vi "UnexpectedDepsCheck.vi"(6 "GUI Mode? {F)":bool, 8 "error in (no error)":errorcluster, 10 "CheckChangedLibrariesOnly":bool=TRUE, 11 "Workspace Path":path=path "C:/sw-deps-monitor") -> (0 "error out":errorcluster, 2 "Status Indicator":string, 3 "Failures":T1[](array[typedef]))   [LabVIEW 2019, in "DepsWatch.lvlib"]
uses:
  DepsWatch.lvlib
  Typedefs/DepsCheckResult.ctl
  28450a76-a9d3-48c7-9439-369bd691228e.vi
  <vilib>/JDP Science/JSONtext/Variant to JSON Text.vi
  <vilib>/Wiresmith Technology/G CLI/CLI Class/CLI.lvclass
  <vilib>/JDP Science/JSONtext/LVClass Serializer/JSONtext LVClass Serializer.lvclass
  <vilib>/SLL Toolkit/SLL String/SLL String.lvlib
  <vilib>/JDP Science/JSONtext/JSONtext.lvlib
panel:
  in  "Tab Control":enum32{"GUI Mode", "CLI Mode"}(tab)
  out "Args":string[](array[string])=["C:\\sw-deps-monitor", "True"]
  # "When in GUI Mode, the controls will be used, \nIn CLI Mode, the Args will be used"
  # "Workspace Path"
  # "CheckChangedLibrariesOnly? True/False"
  # "Command to run the VI from terminal\ng-cli -v --lv-ver 2023 --arch 32 \"C:\\sw-deps-monitor\\CICD\\AutomatedChecks\\UnexpectedDepsCheck.vi\" -- \"C:\\sw-deps-monitor\" \"False\""
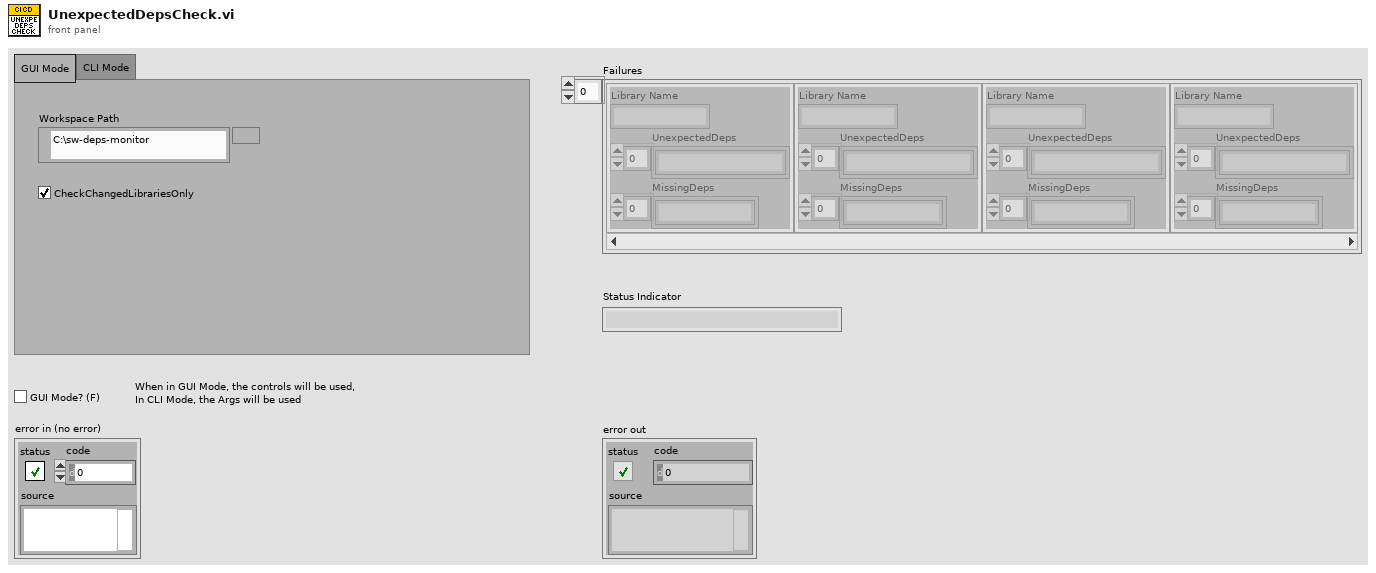
[diagram p1: front panel]
types:
  T1 = typedef "DepsWatch.lvlib/DepsCheckResult.ctl" = cluster{"Library Name":string, "UnexpectedDeps":string[], "MissingDeps":string[]}
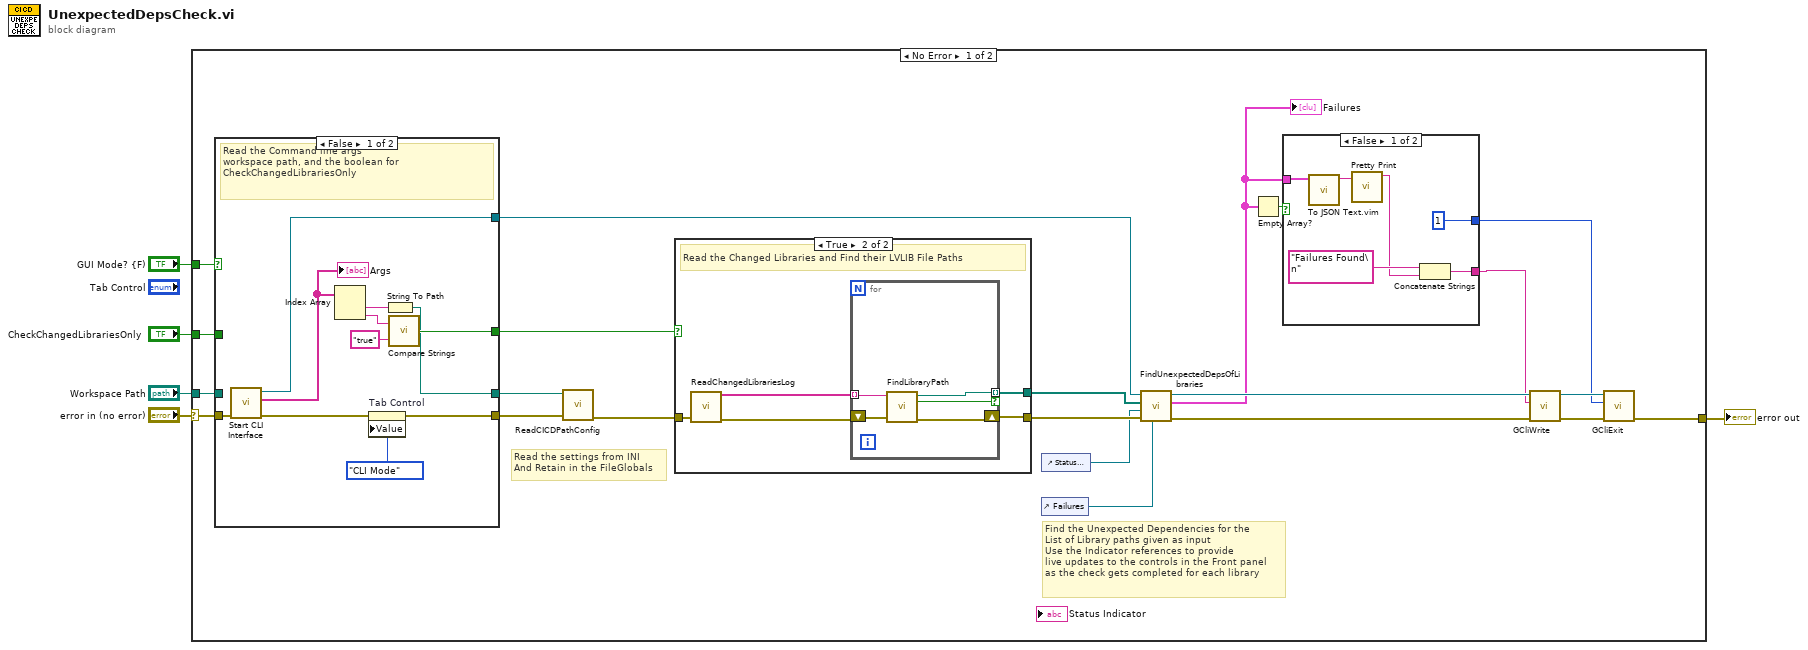
[diagram p0: block diagram]
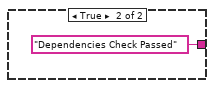
[diagram p2: hidden frame]
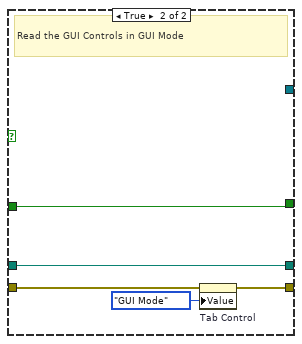
[diagram p3: hidden frame]
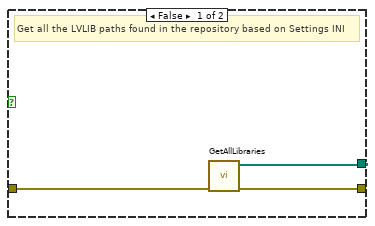
[diagram p4: hidden frame]
diagram:
  n1 = case shown="No Error" "error in (no error)" {
    selector: "error in (no error)" -> [w25 w64]
    tunnel: "GUI Mode? {F)" -> [w26 _]
    tunnel: [w14 w64] -> w3
    tunnel: "CheckChangedLibrariesOnly" -> [w8 _]
    tunnel: "Workspace Path" -> [w7 _]
    frame No Error {
      # "Find the Unexpected Dependencies for the\nList of Library paths given as input\nUse the Indicator references to provide \nlive updates to the controls in the Front panel\nas the check gets completed for each library"
      # "Read the settings from INI\nAnd Retain in the FileGlobals"
      n2 = case shown="False" w26 {
        tunnel: w25 -> [w45 w50]
        tunnel: [w42 w49] -> w23
        tunnel: [w38 w47] -> w24
        tunnel: [w37 w46] -> w22
        tunnel: [w35 _] -> w21
        tunnel: w8 -> [_ w47]
        tunnel: w7 -> [_ w46]
        frame False {
          # "Read the Command line args\nworkspace path, and the boolean for\nCheckChangedLibrariesOnly"
          n3 = call <vilib>:"Start CLI Interface.vi"("error in (no error)"=w45) -> ("error out"=w44:errorcluster, "Custom Parameters"=w36:string[], "CLI out"=w35:refnum<class "CLI.lvclass">)  [unwired: 7 in, 1 out]
          "Args" <- w36
          n4 = Index Array(array=w36) -> (element #1=w41:string, element #2=w40:string)  [unwired: 2 in]
          n5 = property on="Tab Control" class="TabCtl (strict)"(error in=w44, "Value"=enum32{"GUI Mode", "CLI Mode"}."CLI Mode" ("Tab Control")) -> (error out=w42:errorcluster)  [unwired: 1 in, 1 out]
          n6 = String To Path(string=w41) -> (path=w37:path)
          n7 = call <vilib>:"Compare Strings.vi"("y"="true", "x"=w40) -> ("Equal?"=w38:bool)
        }
        frame True {
          # "Read the GUI Controls in GUI Mode"
          n8 = property on="Tab Control" class="TabCtl (strict)"(error in=w50, "Value"=enum32{"GUI Mode", "CLI Mode"}."GUI Mode" ("Tab Control")) -> (error out=w49:errorcluster)  [unwired: 1 in, 1 out]
        }
      }
      n9 = call "ReadCICDPathConfig.vi"("error in (no error)"=w23, "Workspace Path"=w22) -> ("error out"=w27:errorcluster)  [unwired: 8 in, 1 out]
      n10 = case shown="True" w24 {
        tunnel: w27 -> [w51 w56]
        tunnel: [w53 w58] -> w11
        tunnel: [w52 w57] -> w12
        frame False {
          # "Get all the LVLIB paths found in the repository based on Settings INI"
          n11 = call "GetAllLibraries.vi"("error in (no error)"=w51) -> ("error out"=w52:errorcluster, "Lvlib paths"=w53:path[])  [unwired: 9 in]
        }
        frame True {
          # "Read the Changed Libraries and Find their LVLIB File Paths"
          n12 = call "ReadChangedLibrariesLog.vi"("error in (no error)"=w56) -> ("error out"=w55:errorcluster, "ChangedLibraries"=w54:string[])  [unwired: 9 in]
          n13 = for {
            tunnel: w54 -> [w59] mode=indexing
            shift-right: [w62] -> w57
            shift-left: w55 -> [w63]
            tunnel: [w61] -> w58 mode=indexing if=w60
            n14 = call "FindLibraryPath.vi"("error in (no error)"=w63, "Library Name"=w59) -> ("error out"=w62:errorcluster, "Found?"=w60:bool, "Library Path"=w61:path)  [unwired: 7 in]
          }
        }
      }
      n15 = control-ref of="Status Indicator"() -> (w10:refnum<vi>)
      n16 = control-ref of="Failures"() -> (w9:refnum<vi>)
      n17 = call "FindUnexpectedDepsOfLibraries.vi"("Failures Indicator Ref"=w9, "error in (no error)"=w12, "Status Indicator Ref"=w10, "Lvlib paths"=w11, "CLI in"=w21) -> ("error out"=w20:errorcluster, "Failures Array"=w6:T1[], "CLI out"=w18:refnum<class "CLI.lvclass">)  [unwired: 4 in]
      "Failures" <- w6
      n18 = Empty Array?(array=w6) -> (empty?=w16:bool)
      n19 = case shown="False" w16 {
        tunnel: w6 -> [w32 _]
        tunnel: [w31 "Dependencies Check Passed"] -> w15
        tunnel: [1 _] -> w13
        frame False {
          n20 = call "To JSON Text.vim"("Anything"=w32) -> ("<JSON>"=w29:string)  [unwired: 9 in, 1 out]
          n21 = call <vilib>:"Pretty Print.vi"("JSON"=w29) -> ("<JSON>"=w28:string)  [unwired: 8 in, 2 out]
          n22 = Concatenate Strings("Failures Found\n" ("string"), w28) -> (w31:string)
        }
        frame True {
        }
      }
      n23 = call "GCliWrite.vi"("error in (no error)"=w20, "Text to Write"=w15, "CLI in"=w18) -> ("error out"=w19:errorcluster, "CLI out"=w17:refnum<class "CLI.lvclass">)  [unwired: 7 in]
      n24 = call "GCliExit.vi"("error in (no error)"=w19, "No Error Code (0)"=w13, "CLI in"=w17) -> ("error out"=w14:errorcluster)  [unwired: 8 in]
    }
    frame Error {
    }
  }
  "error out" <- w3
